vi "Enable Control.vi"(8 "error in (no error)":errorcluster, 10 "Enable Control":bool, 11 "Lakeshore 331 in":refnum<class "Lakeshore 331.lvclass">) -> (0 "error out":errorcluster, 3 "Lakeshore 331 out":refnum<class "Lakeshore 331.lvclass">)   [LabVIEW 2022 SP3, in "Lakeshore 331.lvclass"]
uses:
  Lakeshore 331.lvclass
  Lakeshore 331.lvclass/Lakeshore 331.ctl
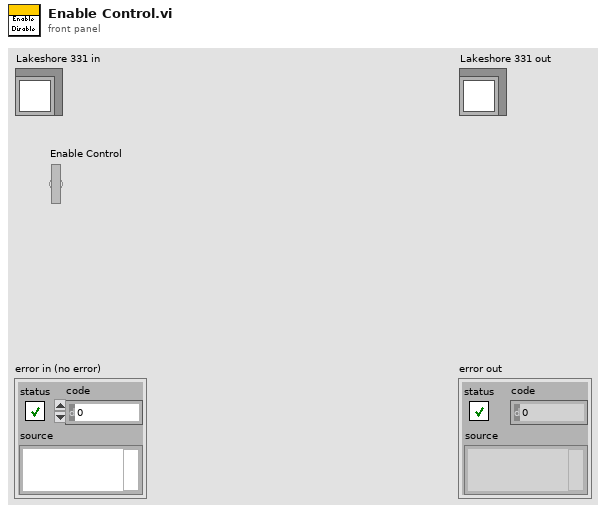
[diagram p1: front panel]
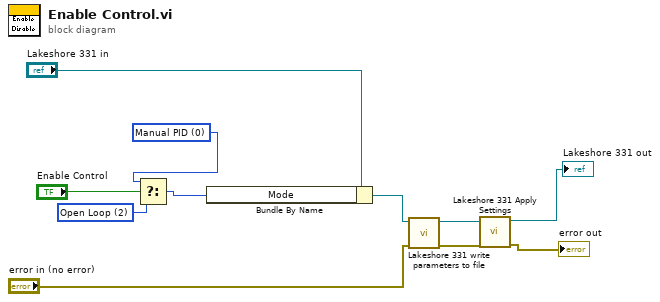
[diagram p0: block diagram]
diagram:
  w9 = u16 2 items=["Manual PID", "Zone", "Open Loop", "AutoTune PID", "AutoTune PI", "AutoTune P"] ("Control Mode (0: Manual PID)")
  w10 = u16 0 items=["Manual PID", "Zone", "Open Loop", "AutoTune PID", "AutoTune PI", "AutoTune P"] ("Control Mode (0: Manual PID)")
  n1 = Select(t=w10, s="Enable Control", f=w9) -> (s? t:f=w8:u16)
  n2 = Bundle By Name(cluster="Lakeshore 331 in", "Mode"=w8) -> (w4:refnum<class "Lakeshore 331.lvclass">)
  n3 = call "Lakeshore 331 write parameters to file.vi"("error in (no error)"="error in (no error)", "Lakeshore 331 in"=w4) -> ("error out"=w5:errorcluster, "Lakeshore 331 out"=w6:refnum<class "Lakeshore 331.lvclass">)  [unwired: 8 in]
  n4 = call "Lakeshore 331 Apply Settings.vi"("error in (no error)"=w5, "Lakeshore 331 in"=w6) -> ("error out"=→"error out":errorcluster, "Lakeshore 331 out"=→"Lakeshore 331 out":refnum<class "Lakeshore 331.lvclass">)  [unwired: 8 in]
